vi "Lightsensor1D.vi"() -> (1 "max index(es)":i32, 2 "max value":dbl)   [LabVIEW 2015]
uses:
  <vilib>/Platform/TimedLoop/XDataNode/timing_clust.ctl
  <vilib>/Platform/TimedLoop/XDataNode/nitl_modes.ctl
  <vilib>/Platform/TimedLoop/XDataNode/wakeup.ctl
  <vilib>/platform/TimedLoop/XDataNode/XDataNode.xnode
  <vilib>/Analysis/NI_AALPro.lvlib
  <vilib>/Platform/TimedLoop/XDataNode/XDNodeRunTimeDep.lvlib
panel:
  out "Array 2":dbl[](array[numeric])
  out "Waveform Graph 2":dbl[](graph)
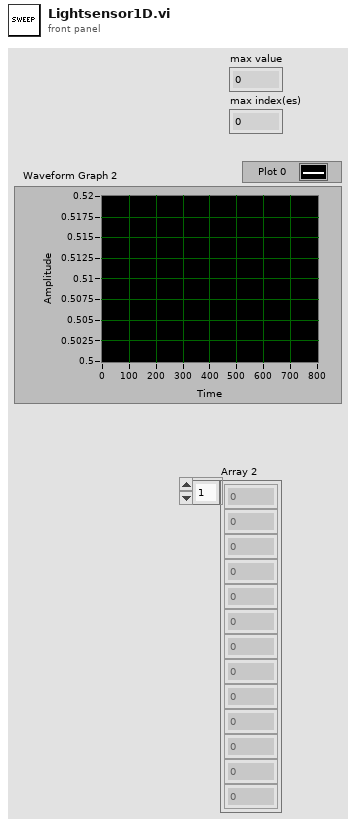
[diagram p1: front panel]
types:
  T1 = typedef "XDNodeRunTimeDep.lvlib/timing_clust.ctl" = cluster{"Expected End [f-1]":u64, "Actual End [f-1]":u64, "Finished Late? [f-1]":bool, "Expected End [i-1]":u64, "Actual End [i-1]":u64, "Finished Late? [i-1]":bool, "Expected Start [i]":u64, "Actual Start [i]":u64, "Expected Start [f]":u64, "Actual Start [f]":u64, "Source Name":string, "Structure Name":string, "Period":i64, "Deadline":i64, "Offset":i64, "Start":i64, "Priority":i32, "Timeout":i32, "Mode":T2, "Wakeup Reason":T3, "Error":errorcluster, "Source Type":string, "Secondary Source Type":string, "Global End Time":u64, "Global Start Time":u64, "Frame Duration":u64, "Iteration Duration":u64, "Assigned CPU":i32, "I/O Scan Engine Mode":u32}
  T2 = typedef "XDNodeRunTimeDep.lvlib/nitl_modes.ctl" = enum32{"No Change", "Process missed periods, maintain original phase", "Discard missed periods, maintain original phase", "Process missed periods, ignore original phase", "Discard missed periods, ignore original phase"}
  T3 = typedef "XDNodeRunTimeDep.lvlib/wakeup.ctl" = enum32{"Normal", "Aborted", "Asynchronous wakeup", "Timing source error", "Timed loop error", "Timeout"}
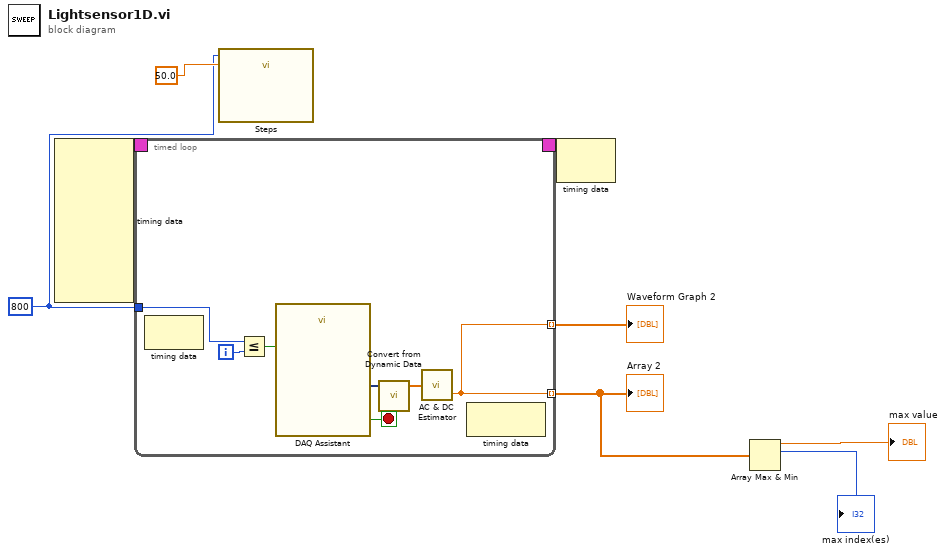
[diagram p0: block diagram]
diagram:
  w1 = 800
  n1 = node-c288() -> (w8:T1)  [unwired: 9 in]
  n2 = timed-loop {
    tunnel: [w13] -> w6 mode=indexing
    tunnel: [w13] -> w5 mode=indexing
    timing: w8 -> [_]
    timing-out: [_] -> w7
    tunnel: w1 -> [w12]
    i -> [w9]
    stop <- w10 stop-if-true
    n3 = node-c288() -> ()  [unwired: 1 in, 1 out]
    n4 = Less Or Equal?(x=w12, y=w9) -> (x <= y?=w11:bool)
    n5 = call "DAQ Assistant"("stop (F)"=w11) -> ("data"=w15:dynamicdata, "stopped"=w10:bool)  [unwired: 15 in, 2 out]
    n6 = call "Convert from Dynamic Data"("Dynamic Data Type"=w15) -> ("Array"=w14:dbl[])  [unwired: 3 in]
    n7 = call <vilib>:"AC & DC Estimator.vi"("Signal (V)"=w14) -> ("DC estimate (V)"=w13:dbl)  [unwired: 1 out]
    n8 = node-c288() -> ()  [unwired: 1 in, 1 out]
  }
  "Waveform Graph 2" <- w6
  "Array 2" <- w5
  n9 = call "Steps"("number of samples"=w1, "timeout (s)"=50.0) -> ()  [unwired: 16 in, 2 out]
  n10 = node-c288(w7) -> ()  [unwired: 1 out]
  n11 = Array Max & Min(array=w5) -> (max value=→"max value":dbl, max index (indices)=→"max index(es)":i32)  [unwired: 2 out]
